vi "test_TCP_1_ Host.vi"() -> ()   [LabVIEW 2014]
panel:
  out "accumRead":string
  out "error out":errorcluster
  out "currentRead":string
  in  "stop":bool
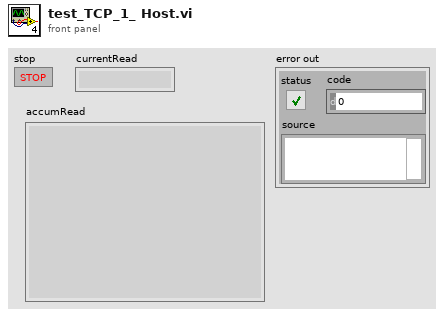
[diagram p1: front panel]
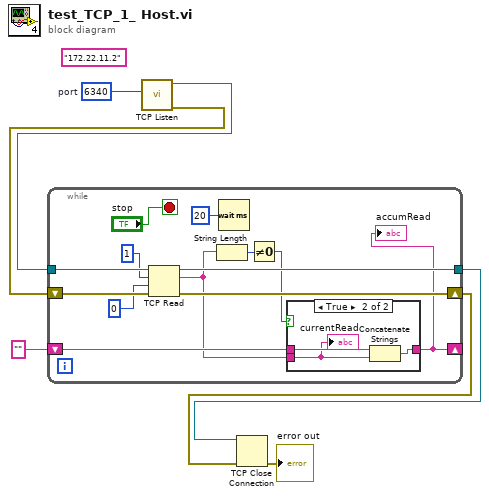
[diagram p0: block diagram]
diagram:
  (unwired) "172.22.11.2" ("address")
  w3 = u16 6340  # port
  n1 = call <vilib>:"TCP Listen.vi"("port"=w3) -> ("error out"=w1:errorcluster, "connection ID"=w2:refnum<k5>)  [unwired: 6 in, 3 out]
  n2 = while {
    tunnel: w2 -> [w18]
    shift-right: [w14] -> w6
    shift-left: w1 -> [w17]
    tunnel: [w13] -> w5
    shift-right: [w8] -> _
    shift-left: "" -> [w10]
    stop <- "stop" stop-if-true
    n3 = TCP Read(connection ID=w18, bytes to read=1, error in (no error)=w17, 9:0 ("timeout ms (25000)")) -> (connection ID out=w13:refnum<k5>, data out=w9:string, error out=w14:errorcluster)  [unwired: 1 out]
    n4 = String Length(string=w9) -> (length=w12:i32)
    n5 = Wait (ms)(milliseconds to wait=u32 20) -> ()  [unwired: 1 out]
    n6 = Not Equal To 0?(x=w12) -> (x != 0?=w11:bool)
    n7 = case shown="True" w11 {
      tunnel: w10 -> [w21 w24]
      tunnel: w9 -> [_ w22]
      tunnel: [w21 w23] -> w8
      frame False {
      }
      frame True {
        n8 = Concatenate Strings(w24, w22) -> (w23:string)
        "currentRead" <- w22
      }
    }
    "accumRead" <- w8
  }
  n9 = TCP Close Connection(connection ID=w5, error in (no error)=w6) -> (error out=→"error out":errorcluster)  [unwired: 2 out]
